vi "Controller_Rumble.vi"(0 "Joystick Refnum Name":string="Pilot Controller", 1 "Rumble":bool) -> ()   [LabVIEW 2018]
uses:
  <vilib>/Rock Robotics/WPI/Utilities/WPI_GetSetVariantRefNum.vi
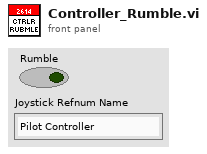
[diagram p1: front panel]
types:
  T1 = typedef "WPI_JoystickDevRef.ctl" = cluster{"Device":T2}
  T2 = typedef "WPI_JoystickDeviceEnum.ctl" = enum16{"USB 0", "USB 1", "USB 2", "USB 3", "USB 4", "USB 5"}
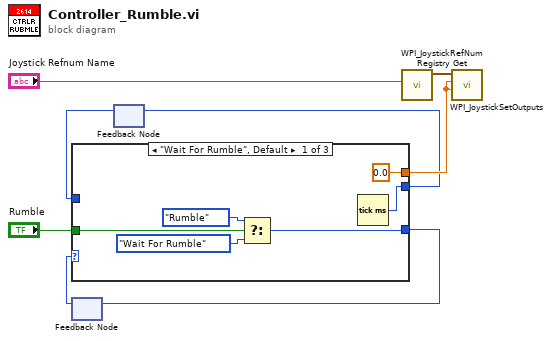
[diagram p0: block diagram]
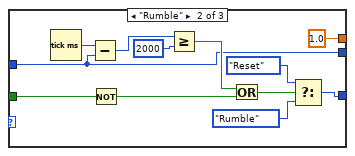
[diagram p2: hidden frame]
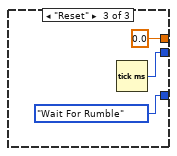
[diagram p3: hidden frame]
diagram:
  n1 = feedback #1() -> (w3:enum16{"Wait For Rumble", "Rumble", "Reset"})  [unwired: 1 in]
  n2 = feedback #2() -> (w5:u32)  [unwired: 1 in]
  n3 = case shown="\"Wait For Rumble\", Default" w3 {
    tunnel: [0.0 1.0 0.0] -> w7
    tunnel: [w13 w21 w29] -> w6
    tunnel: w5 -> [_ w21 _]
    tunnel: [w10 w20 enum16{"Wait For Rumble", "Rumble", "Reset"}."Wait For Rumble" ("f")] -> w4
    tunnel: "Rumble" -> [w9 w16 _]
    frame "Wait For Rumble", Default {
      n4 = Select(t=enum16{"Wait For Rumble", "Rumble", "Reset"}."Rumble" ("Rumble"), s=w9, f=enum16{"Wait For Rumble", "Rumble", "Reset"}."Wait For Rumble") -> (s? t:f=w10:enum16{"Wait For Rumble", "Rumble", "Reset"})
      n5 = Tick Count (ms)() -> (millisecond timer value=w13:u32)
    }
    frame "Rumble" {
      n6 = Tick Count (ms)() -> (millisecond timer value=w25:u32)
      n7 = Subtract(x=w25, y=w21) -> (x-y=w24:u32)
      n8 = Not(x=w16) -> (.not. x?=w15:bool)
      n9 = Greater Or Equal?(x=w24, y=u32 2000) -> (x >= y?=w22:bool)
      n10 = Or(x=w22, y=w15) -> (x .or. y?=w17:bool)
      n11 = Select(t=enum16{"Wait For Rumble", "Rumble", "Reset"}."Reset" ("f"), s=w17, f=enum16{"Wait For Rumble", "Rumble", "Reset"}."Rumble") -> (s? t:f=w20:enum16{"Wait For Rumble", "Rumble", "Reset"})
    }
    frame "Reset" {
      n12 = Tick Count (ms)() -> (millisecond timer value=w29:u32)
    }
  }
  n13 = feedback-in #1(w4) -> ()
  n14 = feedback-in #2(w6) -> ()
  n15 = call <vilib>:"WPI_JoystickRefNum Registry Get.vi"("refnum name"="Joystick Refnum Name") -> ("JoystickDevRef"=w8:T1)  [unwired: 9 in, 1 out]
  n16 = call <vilib>:"WPI_JoystickSetOutputs.vi"("Right Rumble"=w7, "Left Rumble"=w7, "JoystickDevRef"=w8) -> ()  [unwired: 7 in, 2 out]
